vi "Schumann Frequentie Sensor.vi"() -> ()   [LabVIEW 2022 SP3]
uses:
  <vilib>/DAQmx/read.llb/DAQmx Read (Analog 1D Wfm NChan NSamp).vi
  <vilib>/DAQmx/create/channels.llb/DAQmx Create Channel (AI-Voltage-Basic).vi
  <vilib>/DAQmx/configure/timing.llb/DAQmx Timing (Sample Clock).vi
  <vilib>/DAQmx/miscellaneous.llb/DAQmx Fill In Error Info.vi
  <vilib>/Analysis/3filter.llb/Butterworth Filter (DBL).vi
  <vilib>/Utility/file.llb/Write Delimited Spreadsheet (DBL).vi
  <vilib>/Analysis/NI_AALPro.lvlib
  <vilib>/Analysis/NI_AALBase.lvlib
panel:
  in  "tuner":dbl=0.0005
  out "Averaged power spectrum":T1(graph)={0, "df"=0.1220703125, "Power Spectrum (V^2 rms)"=array[8192 elements]}
  out "Duration of current run [minutes]":dbl=0.83485
  out "Milliseconds last cycle":u32=10004
  out "Measurement":waveform(dbl)[](graph)=[{"t0"=timestamp(3745842956.627287 s since 1904-01-01), "dt"=0.0005, "Y"=array[16384 elements], "attributes"=variant("NI_ChannelName"=variant(string "Dev1/ai0"), "NI_UnitDescription"=variant(string "Volts"))}]
  in  "input terminal configuration":i32(ring)=10106 items=["default"=-1, "RSE"=10083, "NRSE"=10078, "Differential"=10106, "Pseudodifferential"=12529]
  in  "Maximum Value":dbl=0.1 format="%0.2f"
  in  "Minimum Value":dbl=-0.1 format="%0.2f"
  in  "Physical Channel":tag="Dev1/ai0"
  in  "Max. freq. to file":dbl=2000.0 format="%.2f"
  in  "Subtract DC?":bool=TRUE
  out "actual sample period (s)":dbl=0.0005 format="%.6f"
  in  "sampling time (s)":dbl=60.0 format="%.2f"
  in  "comment":string="test outdoors Culemborg 6s sampling time freq also in datafile"
  out "file path":path=path "C:/DATA/USB-6009/2022091210.dat"
  out "current cycle":i32=5
  in  "stop program":bool
  in  "save spectrum?":bool=TRUE
  in  "sampling frequency (Hz)":dbl=2000.0 format="%.2f"
  in  "low cutoff frequency (Hz)":dbl=49.0 format="%.4f"
  in  "high cutoff frequency (Hz)":dbl=51.0 format="%.2f"
  in  "filter type":T2(ring)=enum."Bandstop"
  in  "Filtering":bool
  out "?":cluster{i32[], dbl[]}(graph)={[1, 2, 3, 4], [0.17231058873624275, 2.844991077525064e-09, 4.4725994374326006e-09, 1.3661827689300725e-08]}
  out "Beta":dbl=1.3661827689300725e-08 format="%.4e"
  out "Alpha":dbl=4.4725994374326006e-09 format="%.4e"
  out "Theta":dbl=2.844991077525064e-09 format="%.4e"
  out "Delta":dbl=0.17231058873624275 format="%.4e"
  out "Power Spectrum":T1(graph)={0, "df"=0.1220703125, "Power Spectrum (V^2 rms)"=array[8192 elements]}
  out "Filtered Data":dbl[](array[numeric]) format="%.5f"
  # "Delta"
  # "Theta"
  # "Alpha"
  # "Beta"
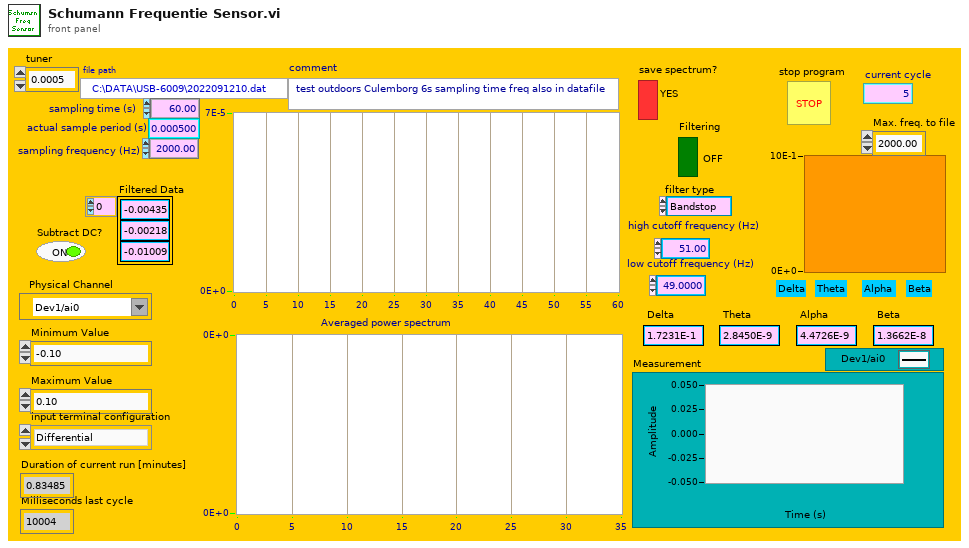
[diagram p1: front panel]
types:
  T1 = cluster{i32, "df":dbl, "Power Spectrum (V^2 rms)":dbl[]}
  T2 = enum32{"Lowpass", "Highpass", "Bandpass", "Bandstop"}
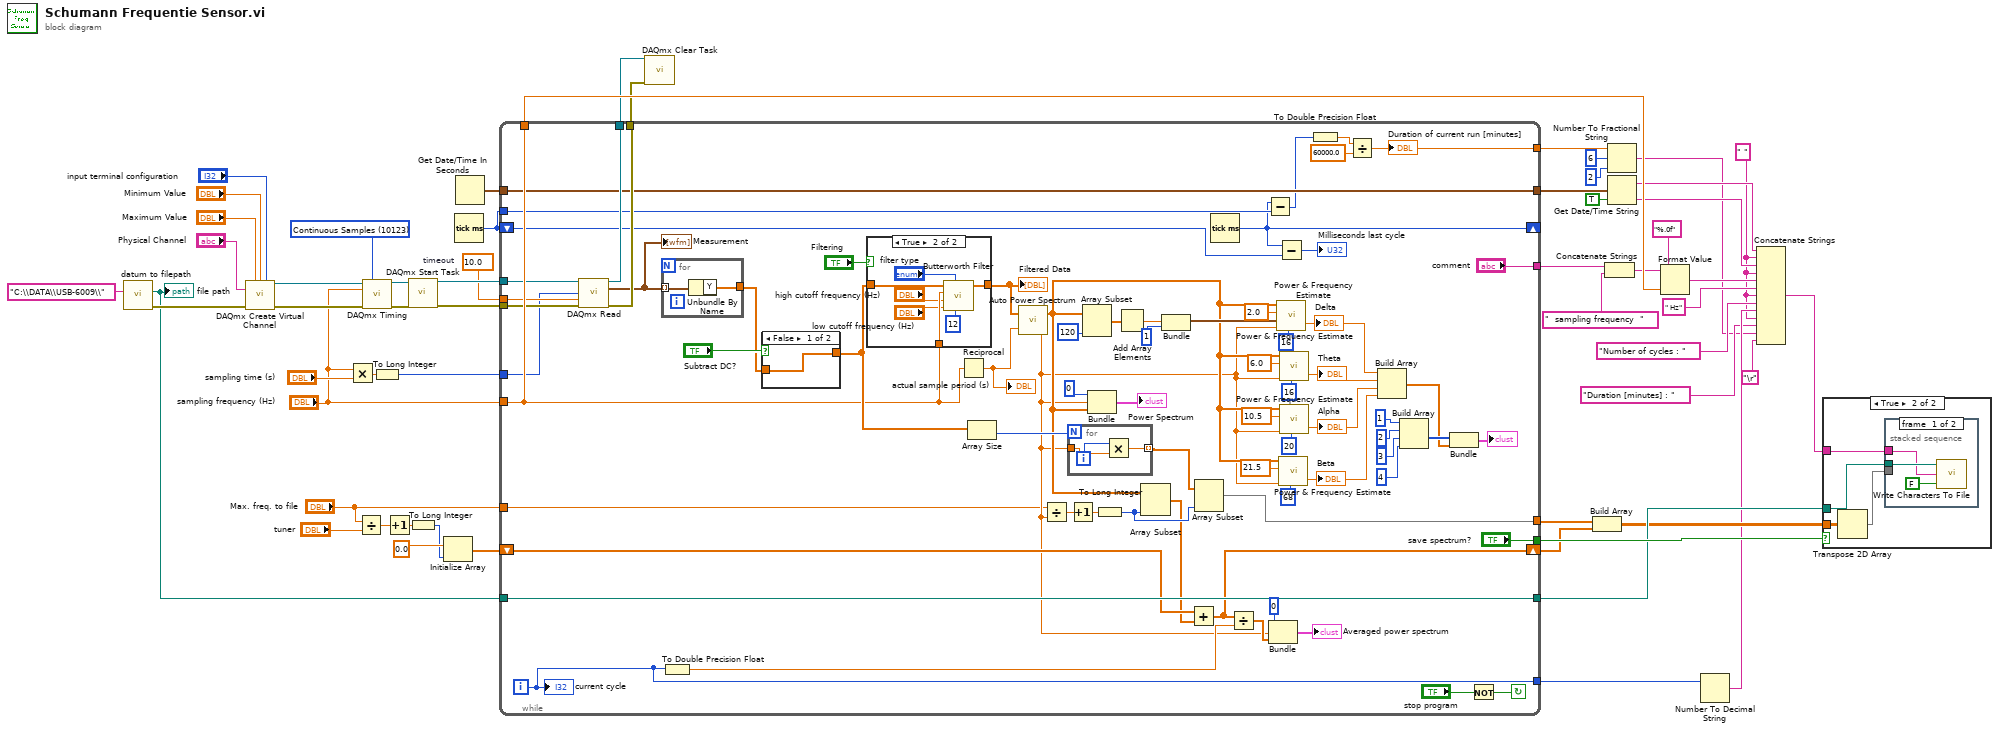
[diagram p0: block diagram]
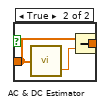
[diagram p2: hidden frame]
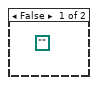
[diagram p4: hidden frame]
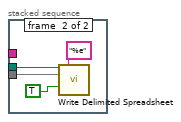
[diagram p5: hidden frame]
diagram:
  w3 = " "
  w35 = 10.0  # timeout
  w46 = 10123 items=["Finite Samples"=10178, "Continuous Samples"=10123] ("sample mode")
  n1 = call "datum to filepath.vi"("prefix"="C:\\DATA\\USB-6009\\") -> ("error out"=w32:errorcluster, "file path"=w31:path)  [unwired: 5 in]
  "file path" <- w31
  n2 = call-poly <vilib>:"DAQmx Create Virtual Channel.vi"("maximum value"="Maximum Value", "minimum value"="Minimum Value", "input terminal configuration"="input terminal configuration", "physical channels"="Physical Channel", "error in"=w32) -> ("task out"=w39:refnum<k21>, "error out"=w40:errorcluster)  [unwired: 9 in]
  n3 = Multiply(x="sampling frequency (Hz)", y="sampling time (s)") -> (x*y=w29:dbl)
  n4 = Divide(x="Max. freq. to file", y="tuner") -> (x/y=w21:dbl)
  n5 = call-poly <vilib>:"DAQmx Timing.vi"("task/channels in"=w39, "sample mode"=w46, "rate"="sampling frequency (Hz)", "error in"=w40) -> ("task out"=w38:refnum<k21>, "error out"=w45:errorcluster)  [unwired: 10 in]
  n6 = To Long Integer(number=w29) -> (32bit integer=w28:i32)
  n7 = Increment(x=w21) -> (x+1=w20:dbl)
  n8 = call <vilib>:"DAQmx Start Task.vi"("task/channels in"=w38, "error in"=w45) -> ("task out"=w37:refnum<k21>, "error out"=w36:errorcluster)  [unwired: 12 in]
  n9 = To Long Integer(number=w20) -> (32bit integer=w19:i32)
  n10 = Initialize Array(0.0, w19) -> (w24:dbl[])
  n11 = Tick Count (ms)() -> (millisecond timer value=w26:u32)
  n12 = Get Date/Time In Seconds() -> (seconds since 1Jan1904=w27:timestamp)
  n13 = while {
    tunnel: [w88] -> w56
    tunnel: ["comment"] -> w51
    tunnel: ["save spectrum?"] -> w57
    tunnel: w31 -> [w96]
    tunnel: [w96] -> w48
    tunnel: "sampling frequency (Hz)" -> [w88]
    tunnel: w37 -> [w86]
    tunnel: w36 -> [w85]
    tunnel: w35 -> [w84]
    tunnel: [w83] -> w34
    tunnel: [w82] -> w33
    tunnel: w28 -> [w79]
    shift-right: [w74] -> _
    shift-left: w26 -> [w78]
    tunnel: w27 -> [w76]
    tunnel: [w76] -> w17
    tunnel: w26 -> [w75]
    shift-right: [w68] -> w12
    shift-left: w24 -> [w71]
    tunnel: "Max. freq. to file" -> [w63]
    tunnel: [w62] -> w13
    tunnel: [w61] -> w9
    tunnel: [w60] -> w7
    i -> [w61]
    stop <- w100 continue-if-true
    n14 = call-poly <vilib>:"DAQmx Read.vi"("task/channels in"=w86, "number of samples per channel"=w79, "timeout"=w84, "error in"=w85) -> ("task out"=w83:refnum<k21>, "data"=w80:waveform(dbl)[], "error out"=w82:errorcluster)  [unwired: 9 in]
    "Measurement" <- w80
    n15 = for {
      tunnel: w80 -> [w130] mode=indexing
      tunnel: [w129] -> w81
      n16 = Unbundle By Name(w130) -> ("Y"=w129:dbl[])
    }
    n17 = To Double Precision Float(number=w61) -> (double precision float=w69:dbl)
    n18 = case shown="False" "Subtract DC?" {
      tunnel: w81 -> [w134 w136]
      tunnel: [w134 w135] -> w94
      frame False {
      }
      frame True {
        n19 = call <vilib>:"AC & DC Estimator.vi"("Signal (V)"=w136) -> ("DC estimate (V)"=w137:dbl)  [unwired: 1 out]
        n20 = Subtract(x=w136, y=w137) -> (x-y=w135:dbl[])
      }
    }
    n21 = case shown="True" "Filtering" {
      tunnel: w94 -> [w138 w144]
      tunnel: [w138 w143] -> w127
      tunnel: w88 -> [_ w142]
      frame False {
      }
      frame True {
        n22 = call-poly <vilib>:"Butterworth Filter.vi"("order"=12, "filter type"="filter type", "low cutoff freq: fl"="low cutoff frequency (Hz)", "high cutoff freq: fh"="high cutoff frequency (Hz)", "sampling freq: fs"=w142, "X"=w144) -> ("Filtered X"=w143:dbl[])  [unwired: 2 in, 1 out]
      }
    }
    "Filtered Data" <- w127
    n23 = Reciprocal(x=w88) -> (1/x=w87:dbl)
    "actual sample period (s)" <- w87
    n24 = Array Size(array=w94) -> (size(s)=w93:i32)
    n25 = call <vilib>:"Auto Power Spectrum.vi"("dt"=w87, "Signal (V)"=w127) -> ("df"=w65:dbl, "Power Spectrum (V^2 rms)"=w90:dbl[])
    n26 = Divide(x=w63, y=w65) -> (x/y=w92:dbl)
    n27 = for {
      N: w93 -> [_]
      tunnel: w65 -> [w133]
      tunnel: [w131] -> w91 mode=indexing
      i -> [w132]
      n28 = Multiply(x=w132, y=w133) -> (x*y=w131:dbl)
    }
    n29 = Increment(x=w92) -> (x+1=w89:dbl)
    n30 = Array Subset(array=w90, length=120) -> (w125:dbl[])  [unwired: 1 in]
    n31 = Bundle(0, "df"=w65, "Power Spectrum (V^2 rms)"=w90) -> (→"Power Spectrum":T1)  [unwired: 1 in]
    n32 = To Long Integer(number=w89) -> (32bit integer=w72:i32)
    n33 = Add Array Elements(numeric array=w125) -> (sum=w124:dbl)
    n34 = Array Subset(array=w90, length=w72) -> (w70:dbl[])  [unwired: 1 in]
    n35 = Bundle(w124, 1) -> (w122:cluster{dbl, i32})  [unwired: 1 in]
    n36 = Add(x=w71, y=w70) -> (x+y=w68:dbl[])
    n37 = Array Subset(array=w91, length=w72) -> (w62:dbl[])  [unwired: 1 in]
    n38 = Tick Count (ms)() -> (millisecond timer value=w74:u32)
    n39 = Divide(x=w68, y=w69) -> (x/y=w66:dbl[])
    n40 = Subtract(x=w74, y=w75) -> (x-y=w59:u32)
    n41 = Bundle(0, "df"=w65, w66) -> (→"Averaged power spectrum":cluster{i32, "df":dbl, dbl[]})  [unwired: 1 in]
    n42 = Subtract(x=w74, y=w78) -> (x-y=→"Milliseconds last cycle":u32)
    n43 = call <vilib>:"Power & Frequency Estimate.vi"("span"=16, "df"=w65, "window constants"=w122, "peak frequency (max)"=2.0, "Power Spectrum (V^2 rms)"=w90) -> ("est power peak"=w119:dbl)  [unwired: 1 in, 1 out]
    "Delta" <- w119
    n44 = call <vilib>:"Power & Frequency Estimate.vi"("span"=68, "df"=w65, "peak frequency (max)"=21.5, "Power Spectrum (V^2 rms)"=w90) -> ("est power peak"=w105:dbl)  [unwired: 2 in, 1 out]
    "Beta" <- w105
    n45 = call <vilib>:"Power & Frequency Estimate.vi"("span"=16, "df"=w65, "peak frequency (max)"=6.0, "Power Spectrum (V^2 rms)"=w90) -> ("est power peak"=w106:dbl)  [unwired: 2 in, 1 out]
    "Theta" <- w106
    n46 = call <vilib>:"Power & Frequency Estimate.vi"("span"=20, "df"=w65, "peak frequency (max)"=10.5, "Power Spectrum (V^2 rms)"=w90) -> ("est power peak"=w112:dbl)  [unwired: 2 in, 1 out]
    "Alpha" <- w112
    n47 = To Double Precision Float(number=w59) -> (double precision float=w58:dbl)
    n48 = Divide(x=w58, y=60000.0) -> (x/y=w60:dbl)
    "Duration of current run [minutes]" <- w60
    n49 = Build Array(w119, w106, w112, w105) -> (w104:dbl[])
    n50 = Build Array(1, 2, 3, 4) -> (w107:i32[])
    n51 = Bundle(w107, w104) -> (→"?":cluster{i32[], dbl[]})  [unwired: 1 in]
    n52 = Not(x="stop program") -> (.not. x?=w100:bool)
    "current cycle" <- w61
  }
  n53 = call <vilib>:"DAQmx Clear Task.vi"("task in"=w34, "error in"=w33) -> ()  [unwired: 13 in, 1 out]
  n54 = Build Array(w13, w12) -> (w11:dbl[][])
  n55 = Concatenate Strings(w51, "  sampling frequency  ") -> (w52:string)
  n56 = Number To Fractional String(number=w7, width (-)=i16 6, precision (6)=i16 2) -> (F-format string=w1:string)  [unwired: 1 in]
  n57 = Get Date/Time String(seconds (now)=w17, want seconds? (F)=TRUE) -> (date string=w15:string, time string=w14:string)  [unwired: 1 in]
  n58 = Format Value(string ("")=w52, format string="%.0f", value (0)=w56) -> (output string=w54:string)
  n59 = Number To Decimal String(number=w9) -> (decimal integer string=w8:string)  [unwired: 1 in]
  n60 = Concatenate Strings(w15, w3, w14, w3, w54, " Hz", w3, "Number of cycles : ", w8, w3, "Duration [minutes] : ", w1, "\r" ("string")) -> (w53:string)
  n61 = case shown="True" w57 {
    tunnel: w11 -> [_ w146]
    tunnel: w53 -> [_ w149]
    tunnel: w48 -> [_ w148]
    frame False {
      (unwired) path ""
    }
    frame True {
      n62 = Transpose 2D Array(2D array=w146) -> (transposed array=w147:dbl[][])
      n63 = stacked-sequence {
        tunnel: w148 -> [w152 w154]
        tunnel: w149 -> [w151 _]
        tunnel: w147 -> [_ w153]
        frame #0 {
          n64 = call <vilib>:"Write Characters To File.vi"("append to file? (new file:F)"=FALSE, "character string"=w151, "file path (dialog if empty)"=w152) -> ()  [unwired: 2 in, 1 out]
        }
        frame #1 {
          n65 = call-poly <vilib>:"Write Delimited Spreadsheet.vi"("file path (dialog if empty)"=w154, "format (%.3f)"="%e", "2D data"=w153, "append to file? (new file:F)"=TRUE) -> ()  [unwired: 10 in, 2 out]
        }
      }
    }
  }
